vi "Modes and States 2016.vi"(2 "Robot Commands":T4) -> (5 "Drive/Climb State":T2, 6 "Ball Gatherer State":T3, 7 "Shooter State":T1)   [LabVIEW 2015]
uses:
  Robot Commands 2016.ctl
  Load SS/Roller State.ctl
  Load SS/Ball Gatherer State.ctl
  Drive SS/Drive Subsystem State.ctl
  Shoot SS/Shooter Control.ctl
  Global Variables/Temp Variables.vi
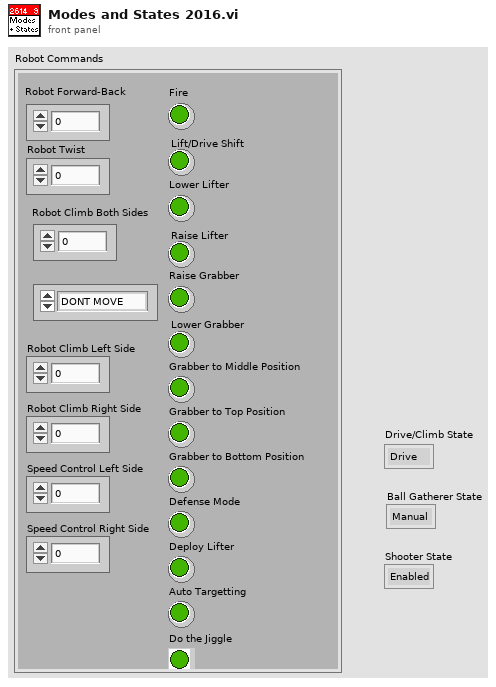
[diagram p1: front panel]
types:
  T1 = typedef "Shooter Control.ctl" = enum16{"Enabled", "Disabled"}
  T2 = typedef "Drive Subsystem State.ctl" = enum16{"Drive", "Climb", "Auto Target"}
  T3 = typedef "Ball Gatherer State.ctl" = enum16{"Manual", "Positional"}
  T4 = typedef "Robot Commands 2016.ctl" = cluster{"Robot Forward-Back":dbl, "Robot Twist":dbl, "Fire":bool, "Lift/Drive Shift":bool, "Raise Lifter":bool, "Raise Grabber":bool, "Lower Grabber":bool, "Roller":T5, "Robot Climb Both Sides":dbl, "Grabber to Middle Position":bool, "Grabber to Top Position":bool, "Grabber to Bottom Position":bool, "Robot Climb Left Side":dbl, "Robot Climb Right Side":dbl, "Speed Control Left Side":dbl, "Speed Control Right Side":dbl, "Lower Lifter":bool, "Defense Mode":bool, "Deploy Lifter":bool, "Auto Targetting":bool, "Do the Jiggle":bool}
  T5 = typedef "Roller State.ctl" = enum16{"DONT MOVE", "Intake", "Outtake"}
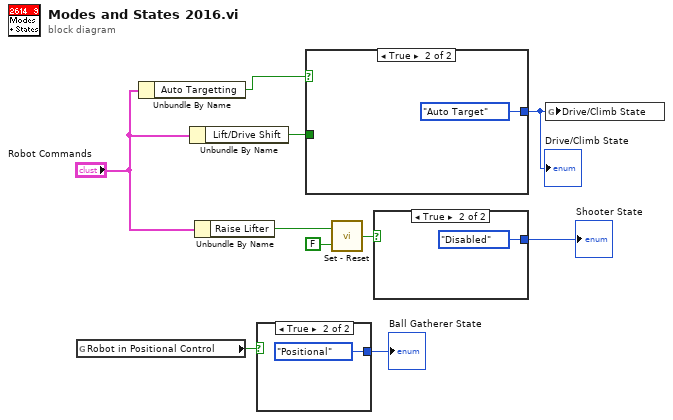
[diagram p0: block diagram]
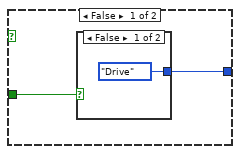
[diagram p2: hidden frame]
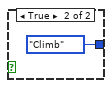
[diagram p3: hidden frame]
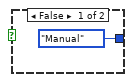
[diagram p4: hidden frame]
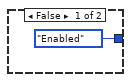
[diagram p5: hidden frame]
diagram:
  n1 = global read "Temp Variables.vi" "Robot in Positional Control"() -> (w2:bool)
  n2 = Unbundle By Name("Robot Commands") -> ("Auto Targetting"=w1:bool)
  n3 = Unbundle By Name("Robot Commands") -> ("Lift/Drive Shift"=w6:bool)
  n4 = Unbundle By Name("Robot Commands") -> ("Raise Lifter"=w10:bool)
  n5 = case shown="True" w2 {
    tunnel: [Ball_Gatherer_State."Manual" ("Ball Gatherer State") Ball_Gatherer_State."Positional" ("Ball Gatherer State")] -> w4
    frame False {
    }
    frame True {
    }
  }
  "Ball Gatherer State" <- w4
  n6 = case shown="True" w1 {
    tunnel: w6 -> [w14 _]
    tunnel: [w13 Drive_Subsystem_State."Auto Target" ("Drive/Climb State")] -> w3
    frame False {
      n7 = case shown="False" w14 {
        tunnel: [Drive_Subsystem_State."Drive" ("Drive/Climb State") Drive_Subsystem_State."Climb" ("Drive/Climb State")] -> w13
        frame False {
        }
        frame True {
        }
      }
    }
    frame True {
    }
  }
  "Drive/Climb State" <- w3
  n8 = call "Set - Reset.vi"("Reset"=FALSE, "Set"=w10) -> ("Output"=w8:bool)
  n9 = case shown="True" w8 {
    tunnel: [Shooter_Control."Enabled" ("Shooter State") Shooter_Control."Disabled" ("Shooter State")] -> w9
    frame False {
    }
    frame True {
    }
  }
  "Shooter State" <- w9
  n10 = global write "Temp Variables.vi" "Drive/Climb State"(w3) -> ()
